vi "RX-SIS-SIM-UDP.vi"(11 "Stop":bool) -> ()   [LabVIEW 2018]
uses:
  <vilib>/Platform/TimedLoop/XDataNode/timing_clust.ctl
  <vilib>/Platform/TimedLoop/XDataNode/nitl_modes.ctl
  <vilib>/Platform/TimedLoop/XDataNode/wakeup.ctl
  Global Variable.vi
  <vilib>/Platform/TimedLoop/XDataNode/XDataNode.xnode
  <vilib>/Platform/TimedLoop/XDataNode/XDNodeRunTimeDep.lvlib
panel:
  out "SIS-SIM-RX-ARRAY":dbl[](array[numeric])
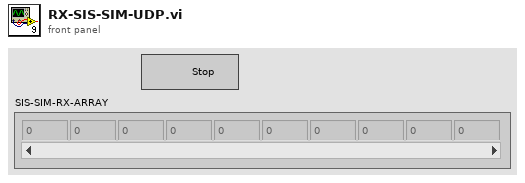
[diagram p1: front panel]
types:
  T1 = typedef "XDNodeRunTimeDep.lvlib/timing_clust.ctl" = cluster{"Expected End [f-1]":u64, "Actual End [f-1]":u64, "Finished Late? [f-1]":bool, "Expected End [i-1]":u64, "Actual End [i-1]":u64, "Finished Late? [i-1]":bool, "Expected Start [i]":u64, "Actual Start [i]":u64, "Expected Start [f]":u64, "Actual Start [f]":u64, "Source Name":string, "Structure Name":string, "Period":i64, "Deadline":i64, "Offset":i64, "Start":i64, "Priority":i32, "Timeout":i32, "Mode":T2, "Wakeup Reason":T3, "Error":errorcluster, "Source Type":string, "Secondary Source Type":string, "Global End Time":u64, "Global Start Time":u64, "Frame Duration":u64, "Iteration Duration":u64, "Assigned CPU":i32, "I/O Scan Engine Mode":u32}
  T2 = typedef "XDNodeRunTimeDep.lvlib/nitl_modes.ctl" = enum32{"No Change", "Process missed periods, maintain original phase", "Discard missed periods, maintain original phase", "Process missed periods, ignore original phase", "Discard missed periods, ignore original phase"}
  T3 = typedef "XDNodeRunTimeDep.lvlib/wakeup.ctl" = enum32{"Normal", "Aborted", "Asynchronous wakeup", "Timing source error", "Timed loop error", "Timeout"}
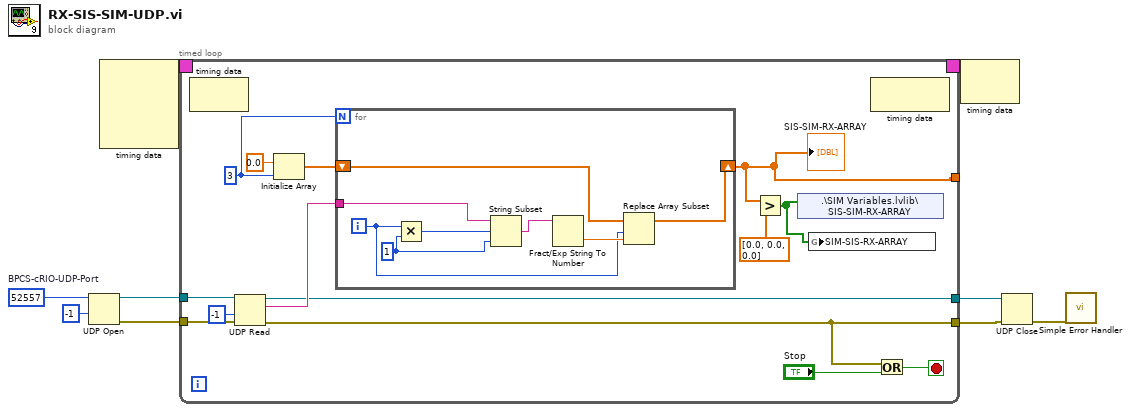
[diagram p0: block diagram]
diagram:
  w7 = u16 52557  # BPCS-cRIO-UDP-Port
  n1 = UDP Open(9:-1 ("timeout ms (25000)"), 11:w7) -> (port=w6:refnum<k16>, 0:w5:errorcluster)  [unwired: 3 in, 1 out]
  n2 = node-c288() -> (w9:T1)  [unwired: 4 in]
  n3 = timed-loop {
    timing: w9 -> [_]
    timing-out: [_] -> w8
    tunnel: w6 -> [w21]
    tunnel: w5 -> [w20]
    tunnel: [w18] -> w3
    tunnel: [w17] -> w2
    tunnel: [w13] -> _
    stop <- w22 stop-if-true
    w14 = 3 ("dimension size")
    n4 = node-c288() -> ()  [unwired: 1 in, 1 out]
    n5 = UDP Read(connection ID=w21, timeout ms (25000)=-1, 8:w20) -> (data out=w19:string, error out=w17:errorcluster, 3:w18:refnum<k16>)  [unwired: 3 out]
    n6 = Initialize Array(0.0 ("element"), w14) -> (w15:dbl[])
    n7 = for {
      N: w14 -> [_]
      tunnel: w19 -> [w30]
      shift-right: [w26] -> w13
      shift-left: w15 -> [w25]
      i -> [w27]
      w24 = 1 ("y")
      n8 = Multiply(x=w27, y=w24) -> (x*y=w29:i32)
      n9 = String Subset(string=w30, offset (0)=w29, length (rest)=w24) -> (substring=w31:string)
      n10 = Fract/Exp String To Number(string=w31) -> (number=w28:dbl)  [unwired: 3 in, 1 out]
      n11 = Replace Array Subset(array=w25, new element=w28, index=w27) -> (w26:dbl[])
    }
    "SIS-SIM-RX-ARRAY" <- w13
    n12 = Greater?(x=w13, y=dbl[] [0.0, 0.0, 0.0]) -> (0:w10:bool[])
    n13 = shared-variable ".\\SIM Variables.lvlib\\SIS-SIM-RX-ARRAY"(w10) -> ()  [unwired: 1 in, 1 out]
    n14 = global write "Global Variable.vi" "SIM-SIS-RX-ARRAY"(w10) -> ()
    n15 = node-c288() -> ()  [unwired: 1 in, 1 out]
    n16 = Or(x=w17, y="Stop") -> (x .or. y?=w22:bool)
  }
  n17 = node-c288(w8) -> ()  [unwired: 1 out]
  n18 = UDP Close(connection ID=w3, 8:w2) -> (error out=w4:errorcluster)  [unwired: 1 out]
  n19 = call <vilib>:"Simple Error Handler.vi"("error in (no error)"=w4) -> ()  [unwired: 4 in, 5 out]
